vi "ROI entry-Event handler-ROI offset.vi"(9 "Offset all ROI-User Event in":refnum<user-event>, 11 "ROI offset arrows: NewVal":T1) -> (0 "error out":errorcluster)   [LabVIEW 2020]
uses:
  Typedefs/Offsets cluster.ctl
  Typedefs/Controls/Multi direction arrows cluster.ctl
  Typedefs/ROI management FG states.ctl
  Globals/gl_ROI Entry UI globals.vi
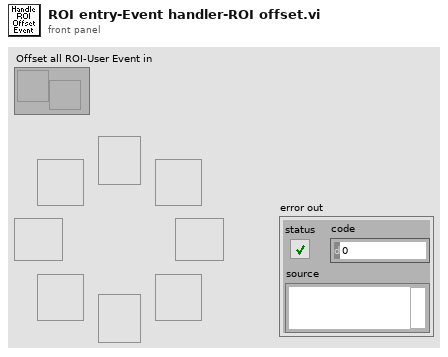
[diagram p1: front panel]
types:
  T1 = typedef "Multi direction arrows cluster.ctl" = cluster{"Right":bool, "Left":bool, "Up":bool, "Down":bool, "Up-left":bool, "Up-right":bool, "Down-left":bool, "Down-right":bool}
  T2 = typedef "ROI management FG states.ctl" = enum16{"Read", "Write", "Write-from dataset", "Clear Last", "Clear All", "Delete ROI", "Update ROIs time", "Reload last ROI set", "Modify ROI Parameters", "Offset all ROI", "Offset visible ROI", "Modify Dwell Time", "Modify Laser Power"}
  T3 = typedef "ROI parameters data type.ctl" = cluster{"ROI index":dbl, "ROI ID":dbl, "ROI Time (ns)":dbl, "Pixels in ROI":dbl, "X start":dbl, "Y start":dbl, "Z start":dbl, "X stop":dbl, "Y stop":dbl, "Z stop":dbl, "Angle (deg)":dbl, "Composite ID":dbl, "Number of lines":dbl, "Frame Size":dbl, "Zoom":dbl, "Laser Power (%)":dbl, "ROI group ID":dbl, "Resolution":dbl, "Dwell Time per pixel":dbl, "Pixels per miniscan":dbl, "Original FOV (um)":dbl, "Apparent Frame Size":dbl, "Z Plane Idx":i32[], "Z Plane codes":i32[]}
  T4 = typedef "Offsets cluster.ctl" = cluster{"X offset":i8, "Y offset":i8}
  T5 = typedef "ROI entry screen ctrl refs cluster.ctl" = cluster{"Done button":refnum<vi>, "Imaging button":refnum<vi>, "Acquisition button":refnum<vi>, "Scan dwell time per pixel (us)":refnum<vi>, "# of planes":refnum<vi>, "Zoom Ctrl":refnum<vi>, "Equal size":refnum<vi>, "Channel":refnum<vi>, "Image Display":refnum<vi>, "Z-Plane Selector":refnum<vi>, "Number of lines left":refnum<vi>, "Z-stack folder path":refnum<vi>, "POI Density":refnum<vi>, "Arb Plane Entry":refnum<vi>, "Whole Plane":refnum<vi>, "Line Mode":refnum<vi>, "Clear Last":refnum<vi>, "Clear All":refnum<vi>, "Delete Lines":refnum<vi>, "Trial Length (sec)":refnum<vi>, "Palette Type":refnum<vi>, "Intensity slider":refnum<vi>, "# POI":refnum<vi>, "Max Z Proj":refnum<vi>, "Zplane ind":refnum<vi>, "Wavelength (nm)":refnum<vi>, "Number of Trials":refnum<vi>, "Funct stim.trig.enable":refnum<vi>, "Funct stim.trig.delay (s)":refnum<vi>, "Line Mode":refnum<vi>, "Step size (µm)":refnum<vi>, "ROI move mode":refnum<vi>, "Cool-down time (s)":refnum<vi>, "Enable cool-down time":refnum<vi>, "Motor Z ind. (um)":refnum<vi>, "AOL Z ind. (um)":refnum<vi>, "Load Reference Image":refnum<vi>, "Rel.  Res.":refnum<vi>, "ROI LIST":refnum<vi>, "Show All":refnum<vi>, "ROI Type":refnum<vi>, "Start Plane":refnum<vi>, "Stop Plane":refnum<vi>, "Offset ROI":refnum<vi>, "Tab Control":refnum<vi>, "Laser Power(%)":refnum<vi>, "Cycle rate":refnum<vi>, "FOV (Ind.)":refnum<vi>, "Frame Size (Ind.)":refnum<vi>, "Resolution (Ind.)":refnum<vi>, "Pixel Density (Ind)":refnum<vi>, "Laser Power (Ind.)":refnum<vi>, "Dwell Time (Ind.)":refnum<vi>, "Adj MC":refnum<vi>}
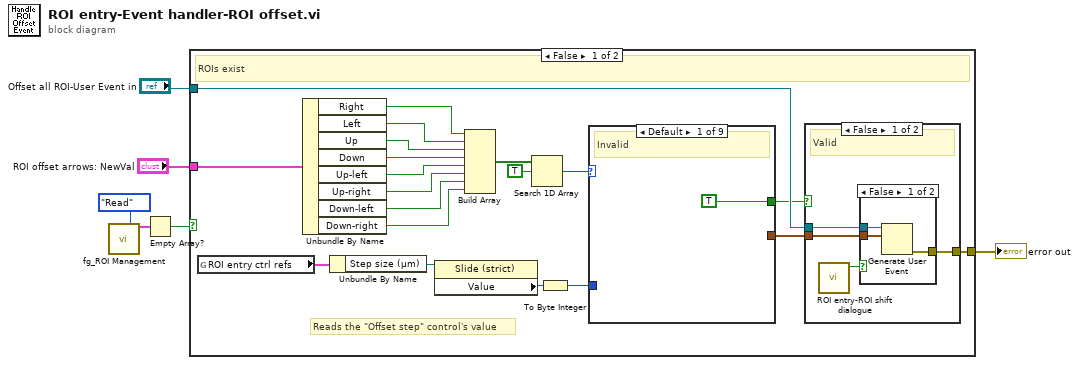
[diagram p0: block diagram]
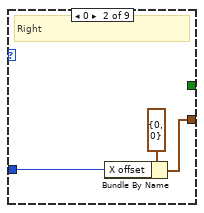
[diagram p4: hidden frame]
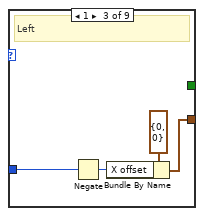
[diagram p5: hidden frame]
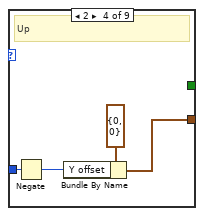
[diagram p6: hidden frame]
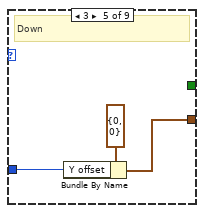
[diagram p7: hidden frame]
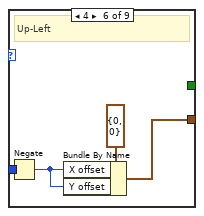
[diagram p8: hidden frame]
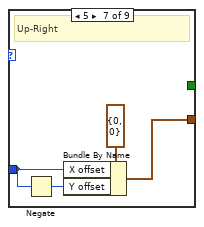
[diagram p9: hidden frame]
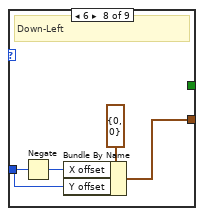
[diagram p10: hidden frame]
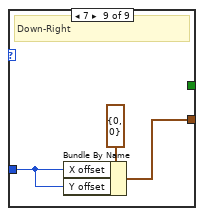
[diagram p11: hidden frame]
diagram:
  n1 = call "fg_ROI Management.vi"("Function"=ROI_management_FG_states."Read") -> ("ROI Setup"=w2:T3[])  [unwired: 8 in, 6 out]
  n2 = Empty Array?(array=w2) -> (empty?=w1:bool)
  n3 = case shown="False" w1 {
    tunnel: [w26 _] -> w6
    tunnel: "Offset all ROI-User Event in" -> [w24 _]
    tunnel: "ROI offset arrows: NewVal" -> [w7 _]
    frame False {
      # "Reads the \"Offset step\" control's value"
      # "ROIs exist"
      n4 = global read "gl_ROI Entry UI globals.vi" "ROI entry ctrl refs"() -> (w11:T5)
      n5 = Unbundle By Name(w7) -> ("Right"=w12:bool, "Left"=w13:bool, "Up"=w14:bool, "Down"=w15:bool, "Up-left"=w16:bool, "Up-right"=w17:bool, "Down-left"=w18:bool, "Down-right"=w19:bool)
      n6 = Unbundle By Name(w11) -> ("Step size (µm)"=w10:refnum<vi>)
      n7 = property class="Slide (strict)"(reference=w10) -> ("Value"=w9:u8)  [unwired: 1 in, 2 out]
      n8 = Build Array(w12, w13, w14, w15, w16, w17, w18, w19) -> (w20:bool[])
      n9 = Search 1D Array(1D array=w20, element=TRUE) -> (index of element=w22:i32)  [unwired: 1 in]
      n10 = To Byte Integer(number=w9) -> (8bit integer=w8:i8)
      n11 = case shown="Default" w22 {
        tunnel: [TRUE _ _ _ _ _ _ _ _] -> w23
        tunnel: [_ w36 w40 w44 w47 w51 w55 w59 w62] -> w25
        tunnel: w8 -> [_ w35 w38 w42 w46 w50 w53 w58 w61]
        frame Default {
          # "Invalid"
        }
        frame 0 {
          # "Right"
          n12 = Bundle By Name(cluster=T4 {"X offset"=0, "Y offset"=0} ("event data"), "X offset"=w35) -> (w36:T4)
        }
        frame 1 {
          # "Left"
          n13 = Negate(x=w38) -> (-x=w39:i8)
          n14 = Bundle By Name(cluster=T4 {"X offset"=0, "Y offset"=0} ("event data"), "X offset"=w39) -> (w40:T4)
        }
        frame 2 {
          # "Up"
          n15 = Negate(x=w42) -> (-x=w43:i8)
          n16 = Bundle By Name(cluster=T4 {"X offset"=0, "Y offset"=0} ("event data"), "Y offset"=w43) -> (w44:T4)
        }
        frame 3 {
          # "Down"
          n17 = Bundle By Name(cluster=T4 {"X offset"=0, "Y offset"=0} ("event data"), "Y offset"=w46) -> (w47:T4)
        }
        frame 4 {
          # "Up-Left"
          n18 = Negate(x=w50) -> (-x=w49:i8)
          n19 = Bundle By Name(cluster=T4 {"X offset"=0, "Y offset"=0} ("event data"), "X offset"=w49, "Y offset"=w49) -> (w51:T4)
        }
        frame 5 {
          # "Up-Right"
          n20 = Negate(x=w53) -> (-x=w54:i8)
          n21 = Bundle By Name(cluster=T4 {"X offset"=0, "Y offset"=0} ("event data"), "X offset"=w53, "Y offset"=w54) -> (w55:T4)
        }
        frame 6 {
          # "Down-Left"
          n22 = Negate(x=w58) -> (-x=w57:i8)
          n23 = Bundle By Name(cluster=T4 {"X offset"=0, "Y offset"=0} ("event data"), "X offset"=w57, "Y offset"=w58) -> (w59:T4)
        }
        frame 7 {
          # "Down-Right"
          n24 = Bundle By Name(cluster=T4 {"X offset"=0, "Y offset"=0} ("event data"), "X offset"=w61, "Y offset"=w61) -> (w62:T4)
        }
      }
      n25 = case shown="False" w23 {
        tunnel: w24 -> [w30 _]
        tunnel: w25 -> [w29 _]
        tunnel: [w28 _] -> w26
        frame False {
          # "Valid"
          n26 = call "ROI entry-ROI shift dialogue.vi"() -> ("Cancelled (Left button pressed)"=w27:bool)  [unwired: 11 in]
          n27 = case shown="False" w27 {
            tunnel: w30 -> [w33 _]
            tunnel: w29 -> [w32 _]
            tunnel: [w31 _] -> w28
            frame False {
              n28 = Generate User Event(user event=w33, event data cluster=w32) -> (error out=w31:errorcluster)  [unwired: 2 in, 1 out]
            }
            frame True {
            }
          }
        }
        frame True {
          # "Invalid"
        }
      }
    }
    frame True {
      # "No ROIs exist"
    }
  }
  "error out" <- w6
